vi "DB_LeeVIF_Graficas.vi"(8 "error in (no error)":errorcluster, 11 "ID_EQUIPO":i32=1) -> (0 "error out":errorcluster, 3 "output cluster":T1)   [LabVIEW 2018]
uses:
  Controls/VIF_cluster.ctl
  <vilib>/addons/database/Connection.llb/DB Tools Open Connec (Path).vi
  <vilib>/addons/database/Connection.llb/Conn Execute.vi
  <vilib>/addons/database/Recordset.llb/Rec Fetch Recordset Data (R).vi
  <vilib>/addons/database/Recordset.llb/Rec Destroy - Connection.vi
  <vilib>/addons/database/_DB Variant To Data/Database Variant To Data.xnode
  <vilib>/addons/database/NI_Database_API.lvlib
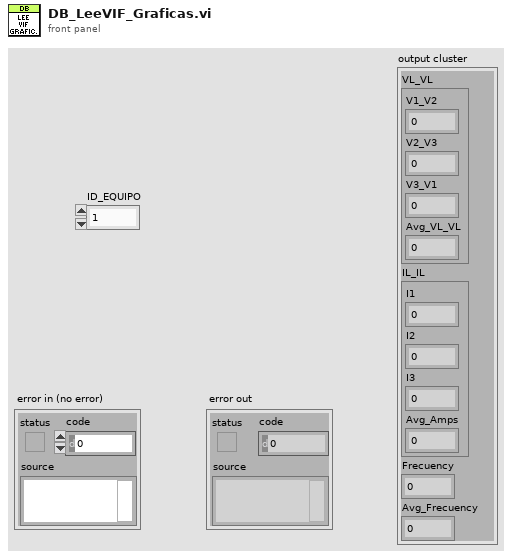
[diagram p1: front panel]
types:
  T1 = typedef "VIF_cluster.ctl" = cluster{"VL_VL":cluster{"V1_V2":sgl, "V2_V3":sgl, "V3_V1":sgl, "Avg_VL_VL":sgl}, "IL_IL":cluster{"I1":sgl, "I2":sgl, "I3":sgl, "Avg_Amps":sgl}, "Frecuency":sgl, "Avg_Frecuency":sgl}
  T2 = cluster{"I1":sgl, "I2":sgl, "I3":sgl, "Avg_Amps":sgl}
  T3 = cluster{"V1_V2":sgl, "V2_V3":sgl, "V3_V1":sgl, "Avg_VL_VL":sgl}
  T4 = typedef "NI_Database_API.lvlib/Conn ObjectReference.ctl" = refnum<k1>
  T5 = typedef "NI_Database_API.lvlib/Rec ObjectReference.ctl" = refnum<k1>
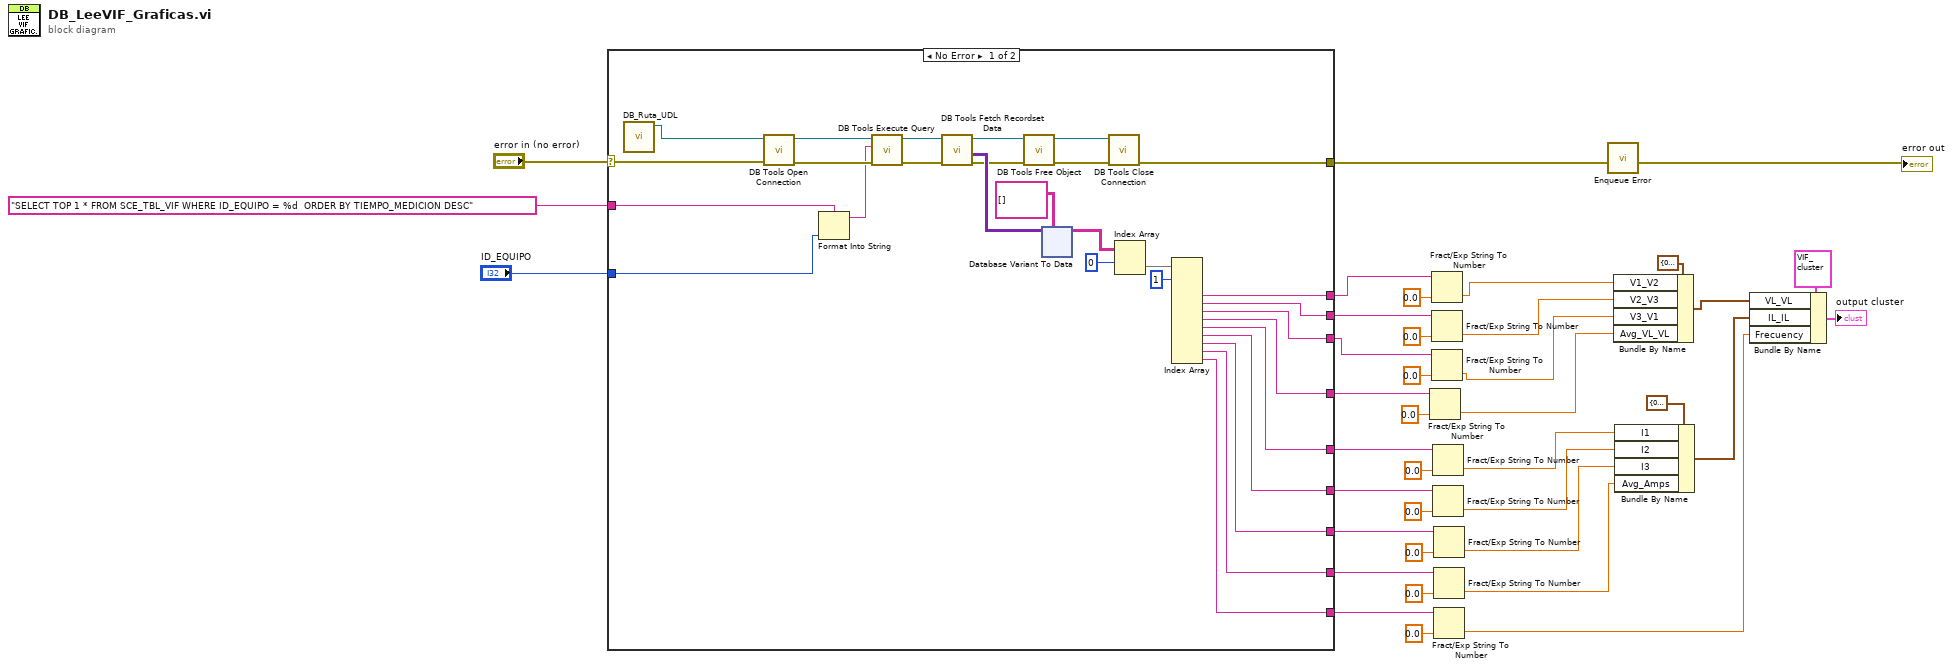
[diagram p0: block diagram]
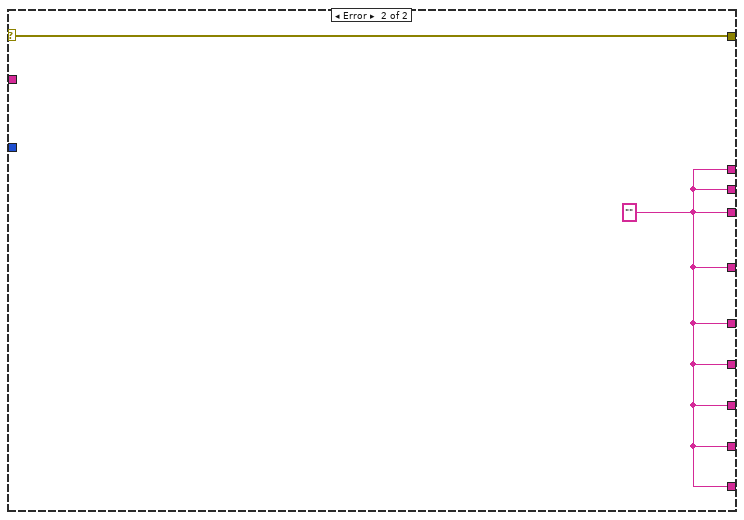
[diagram p2: hidden frame]
diagram:
  n1 = case shown="No Error" "error in (no error)" {
    selector: "error in (no error)" -> [w62 w113]
    tunnel: [w64 w113] -> w36
    tunnel: "SELECT TOP 1 * FROM SCE_TBL_VIF WHERE ID_EQUIPO = %d  ORDER BY TIEMPO_MEDICION DESC" ("SQL") -> [w54 _]
    tunnel: [w50 w112] -> w34
    tunnel: [w49 w112] -> w30
    tunnel: [w48 w112] -> w29
    tunnel: "ID_EQUIPO" -> [w51 _]
    tunnel: [w46 w112] -> w25
    tunnel: [w47 w112] -> w24
    tunnel: [w45 w112] -> w23
    tunnel: [w44 w112] -> w21
    tunnel: [w42 w112] -> w6
    tunnel: [w41 w112] -> w4
    frame No Error {
      n2 = call "DB_Ruta_UDL.vi"() -> ("UDL ruta"=w40:path)  [unwired: 11 in]
      n3 = call-poly <vilib>:"DB Tools Open Connection.vi"("error in (no error)"=w62, "connection information"=w40) -> ("error out"=w67:errorcluster, "connection reference"=w65:T4)  [unwired: 6 in]
      n4 = Format Into String(format string=w54, w51) -> (resulting string=w53:string)  [unwired: 2 in, 1 out]
      n5 = call-poly <vilib>:"DB Tools Execute Query.vi"("error in (no error)"=w67, "SQL query"=w53, "connection reference"=w65) -> ("error out"=w63:errorcluster, "recordset reference"=w61:T5)  [unwired: 5 in]
      n6 = call-poly <vilib>:"DB Tools Fetch Recordset Data.vi"("error in (no error)"=w63, "recordset reference"=w61) -> ("error out"=w57:errorcluster, "recordset data"=w58:variant[][], "recordset reference out"=w60:T5)  [unwired: 3 in]
      n7 = call-poly <vilib>:"DB Tools Free Object.vi"("error in (no error)"=w57, "recordset reference"=w60) -> ("error out"=w66:errorcluster, "connection reference"=w39:T4)  [unwired: 8 in]
      n8 = xnode "Database Variant To Data"("database variant"=w58, "type"=string[][] []) -> ("data"=w56:string[][])  [unwired: 1 in, 1 out]
      n9 = call <vilib>:"DB Tools Close Connection.vi"("error in (no error)"=w66, "connection reference"=w39) -> ("error out"=w64:errorcluster)  [unwired: 5 in]
      n10 = Index Array(array=w56, index (row)=0 ("disabled index (col)")) -> (element=w52:string[])  [unwired: 1 in]
      n11 = Index Array(array=w52, index #1=1 ("index")) -> (element #3=w50:string, element #4=w49:string, element #5=w48:string, element #6=w42:string, element #7=w46:string, element #8=w47:string, element #9=w45:string, element #10=w41:string, element #11=w44:string)  [unwired: 10 in, 2 out]
    }
    frame Error {
      w112 = ""
    }
  }
  n12 = Fract/Exp String To Number(string=w6, default (0 dbl)=sgl 0.0) -> (number=w2:sgl)  [unwired: 2 in, 1 out]
  n13 = Fract/Exp String To Number(string=w34, default (0 dbl)=sgl 0.0) -> (number=w17:sgl)  [unwired: 2 in, 1 out]
  n14 = Fract/Exp String To Number(string=w30, default (0 dbl)=sgl 0.0) -> (number=w16:sgl)  [unwired: 2 in, 1 out]
  n15 = Fract/Exp String To Number(string=w29, default (0 dbl)=sgl 0.0) -> (number=w15:sgl)  [unwired: 2 in, 1 out]
  n16 = Fract/Exp String To Number(string=w25, default (0 dbl)=sgl 0.0) -> (number=w13:sgl)  [unwired: 2 in, 1 out]
  n17 = Fract/Exp String To Number(string=w24, default (0 dbl)=sgl 0.0) -> (number=w12:sgl)  [unwired: 2 in, 1 out]
  n18 = Fract/Exp String To Number(string=w23, default (0 dbl)=sgl 0.0) -> (number=w11:sgl)  [unwired: 2 in, 1 out]
  n19 = Fract/Exp String To Number(string=w4, default (0 dbl)=sgl 0.0) -> (number=w3:sgl)  [unwired: 2 in, 1 out]
  n20 = Fract/Exp String To Number(string=w21, default (0 dbl)=sgl 0.0) -> (number=w9:sgl)  [unwired: 2 in, 1 out]
  n21 = call "Enqueue Error.vi"("error in"=w36) -> ("error out"=→"error out":errorcluster)  [unwired: 9 in, 1 out]
  n22 = Bundle By Name(cluster=T3 {"V1_V2"=0.0, "V2_V3"=0.0, "V3_V1"=0.0, "Avg_VL_VL"=0.0} ("VL_VL"), "V1_V2"=w17, "V2_V3"=w16, "V3_V1"=w15, "Avg_VL_VL"=w2) -> (w18:T3)
  n23 = Bundle By Name(cluster=T2 {"I1"=0.0, "I2"=0.0, "I3"=0.0, "Avg_Amps"=0.0} ("IL_IL"), "I1"=w13, "I2"=w12, "I3"=w11, "Avg_Amps"=w3) -> (w10:T2)
  n24 = Bundle By Name(cluster=T1 {"VL_VL"={"V1_V2"=0.0, "V2_V3"=0.0, "V3_V1"=0.0, "Avg_VL_VL"=0.0}, "IL_IL"={"I1"=0.0, "I2"=0.0, "I3"=0.0, "Avg_Amps"=0.0}, "Frecuency"=0.0, "Avg_Frecuency"=0.0} ("VIF_cluster"), "VL_VL"=w18, "IL_IL"=w10, "Frecuency"=w9) -> (→"output cluster":T1)
